vi "Macro Start Release.vi"(7 "tag prefix (level1/level2)":string, 8 "error in (no error)":errorcluster, 10 "VIPB Path":path, 11 "Git in":refnum<class "Git.lvclass">) -> (0 "error out":errorcluster, 3 "Git out":refnum<class "Git.lvclass">)   [LabVIEW 2019, in "Git.lvclass"]
uses:
  Git.lvclass
  Git.lvclass/Git.ctl
  <vilib>/Hampel Software Engineering/Git API/Git API/GIT-api.lvclass
  <vilib>/JKI/VIPM API/VIPM API_vipm_api.lvlib
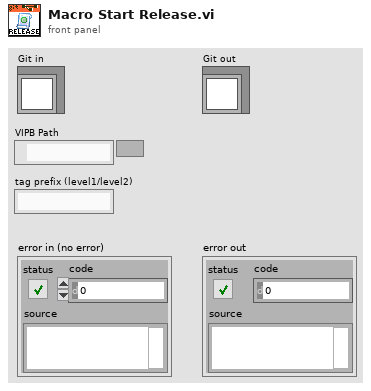
[diagram p1: front panel]
types:
  T1 = typedef "VIPM API_vipm_api.lvlib/VI Package Build Spec Data Cluster_vipm_api.ctl" = cluster{"Package Version":T2, "Product Name":string, "Company Name":string, "Author Name (Person or Company)":string, "Product Homepage (URL)":string, "Legal Copyright":string, "License Agreement Name":string, "Product Description Summary":string, "Product Description":string, "Release Notes - Change Log":string}
  T2 = typedef "VIPM API_vipm_api.lvlib/Version Info Cluster_vipm_api.ctl" = cluster{"major":u32, "minor":u32, "patch":u32, "build":u32}
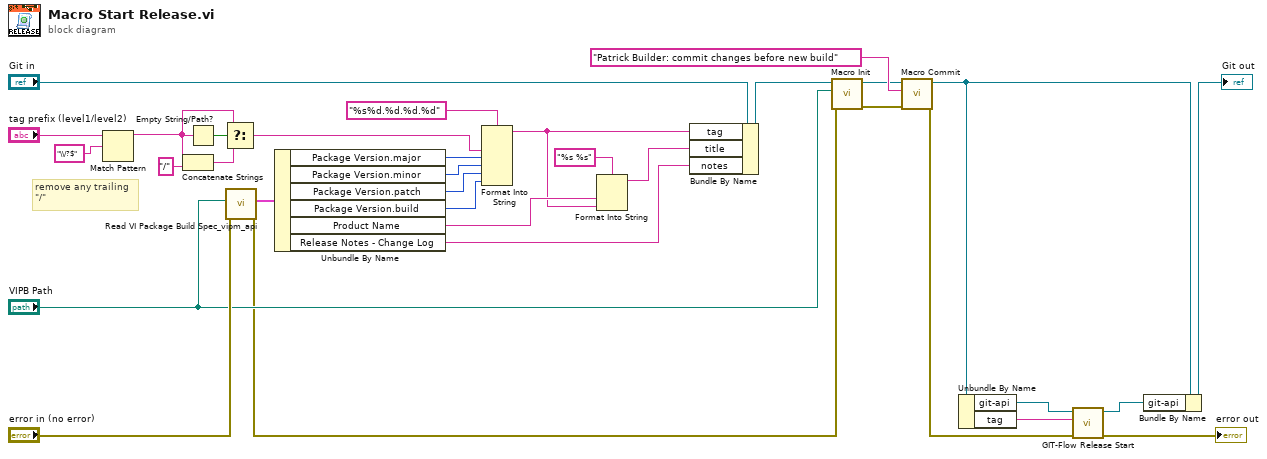
[diagram p0: block diagram]
diagram:
  # "remove any trailing\n\"/\""
  n1 = Match Pattern(string="tag prefix (level1/level2)", regular expression="\\/?$") -> (before substring=w8:string)  [unwired: 1 in, 3 out]
  n2 = Concatenate Strings(w8, "/" ("string")) -> (w11:string)
  n3 = Empty String/Path?(string/path=w8) -> (empty?=w14:bool)
  n4 = Select(t=w8, s=w14, f=w11) -> (s? t:f=w13:string)
  n5 = call <vilib>:"Read VI Package Build Spec_vipm_api.vi"("error in (no error)"="error in (no error)", "Path to VIPB File"="VIPB Path") -> ("error out"=w15:errorcluster, "VI Package Build Spec Data"=w27:T1)  [unwired: 8 in]
  n6 = Unbundle By Name(w27) -> ("Package Version.major"=w20:u32, "Package Version.minor"=w30:u32, "Package Version.patch"=w29:u32, "Package Version.build"=w28:u32, "Product Name"=w23:string, "Release Notes - Change Log"=w19:string)
  n7 = Format Into String(format string="%s%d.%d.%d.%d", w13, w20, w30, w29, w28) -> (resulting string=w22:string)  [unwired: 2 in, 1 out]
  n8 = Format Into String(format string="%s %s", w23, w22) -> (resulting string=w21:string)  [unwired: 2 in, 1 out]
  n9 = Bundle By Name(cluster="Git in", "tag"=w22, "title"=w21, "notes"=w19) -> (w17:refnum<class "Git.lvclass">)
  n10 = call "Macro Init.vi"("error in (no error)"=w15, "Repository Path"="VIPB Path", "Git in"=w17) -> ("error out"=w6:errorcluster, "Git out"=w4:refnum<class "Git.lvclass">)  [unwired: 7 in]
  n11 = call "Macro Commit.vi"("error in (no error)"=w6, "msg"="Patrick Builder: commit changes before new build", "Git in"=w4) -> ("error out"=w5:errorcluster, "Git out"=w3:refnum<class "Git.lvclass">)  [unwired: 7 in]
  n12 = Unbundle By Name(w3) -> ("git-api"=w1:refnum<class "GIT-api.lvclass">, "tag"=w7:string)
  n13 = call <vilib>:"GIT-Flow Release Start.vi"("error in"=w5, "release name"=w7, "Git-API in"=w1) -> ("error out"=→"error out":errorcluster, "Git-API out"=w2:refnum<class "GIT-api.lvclass">)  [unwired: 7 in]
  n14 = Bundle By Name(cluster=w3, "git-api"=w2) -> (→"Git out":refnum<class "Git.lvclass">)
